vi "Wait on Integer Runtime Test.vi"() -> ()   [LabVIEW 2015, in "Wait on Integer Tests.lvlib"]
uses:
  Wait on Integer Tests.lvlib
  Config/Wait On Integer Config.lvclass
  classes/Step/Execution/StepState.ctl
  classes/Step/Execution/Step Status.ctl
  classes/Step/Execution/Step Flow Control.ctl
  <vilib>/NI/Tag Bus/tag/Data Type.ctl
  <vilib>/NI/Tag Bus Module Framework/channel/channel classification.ctl
  Config/Wait On Integer Config.lvclass/Wait On Integer Config.ctl
  <vilib>/NI/Tag Bus/tag/tag descriptor.lvclass/tag descriptor.ctl
  <vilib>/NI/Tag Bus/table/data polymorphs/write one/write U32.vi
  Config/Write Wait On Integer Event.vi
  Config/Write Target Integer.vi
  Config/Write Timeout.vi
  <vilib>/NI/Tag Bus/tag/read tag name.vi
  <vilib>/NI/Tag Bus/tag/read data type.vi
  <vilib>/NI/Tag Bus/dictionary/locate tag.vi
  classes/Step/Execution/Step.lvclass
  <vilib>/NI/Tag Bus Module Framework/channel/TBM channel.lvclass
  <vilib>/NI/Tag Bus/table/data table.lvlib
  <vilib>/NI/Tag Bus/dictionary/data dictionary.lvclass
  <vilib>/NI/Tag Bus/tag/tag descriptor.lvclass
panel:
  out "error out":errorcluster
  in  "Current Integer":u32
  out "Results":bool[](array[boolean])
  in  "Timeout":i32
  in  "Target Integer":i32
  # "Step State\n\nFlow Control\n\nJump Index\n\nDone"
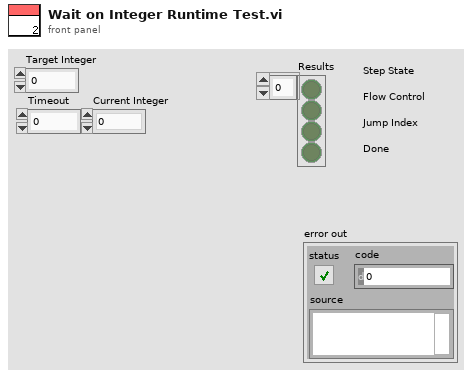
[diagram p1: front panel]
types:
  T1 = typedef "TBM channel.lvclass/channel classification.ctl" = enum16{"input data", "output data", "processing parameter", "processing result"}
  T2 = typedef "tag bus.lvlib/tag descriptor.lvclass/Data Type.ctl" = enum16{"Double", "Single", "I64", "I32", "I16", "I8", "U64", "U32", "U16", "U8", "Boolean", "String", "Array of Double", "Array of Single", "Array of I64", "Array of I32", "Array of I16", "Array of I8", "Array of U64", "Array of U32", "Array of U16", "Array of U8", "Array of Boolean", "Array of String"}
  T3 = typedef "Step.lvclass/Step Status.ctl" = enum16{"Start", "Passed", "Failed", "Error", "Done", "Terminated", "Skipped", "Running"}
  T4 = typedef "Step.lvclass/StepState.ctl" = cluster{"Step State":T3, "Flow Control":T5, "Jump Index":i32, "Done":bool}
  T5 = typedef "Step.lvclass/Step Flow Control.ctl" = enum16{"Next Step", "Jump"}
  T6 = typedef "TBM channel.lvclass/data tables.ctl" = cluster{"input data":T7, "processing parameter":T7, "processing result":T7, "output data":T7}
  T7 = typedef "tag bus.lvlib/dictionary table pair.ctl" = cluster{"data dictionary":refnum<class "data dictionary.lvclass">, "data table":T8}
  T8 = typedef "tag bus.lvlib/data table.lvlib/data table.ctl" = cluster{"Double":dbl[], "Single":sgl[], "I64":i64[], "I32":i32[], "I16":i16[], "I8":i8[], "U64":u64[], "U32":u32[], "U16":u16[], "U8":u8[], "Boolean":bool[], "String":string[], "Array of Double":cluster{"DBL Array":dbl[]}[], "Array of Single":cluster{"SGL Array":sgl[]}[], "Array of I64":cluster{"I64 Array":i64[]}[], "Array of I32":cluster{"I32 Array":i32[]}[], "Array of I16":cluster{"I16 Array":i16[]}[], "Array of I8":cluster{"I8 Array":i8[]}[], "Array of U64":cluster{"U64 Array":u64[]}[], "Array of U32":cluster{"U32 Array":u32[]}[], "Array of U16":cluster{"U16 Array":u16[]}[], "Array of U8":cluster{"U8 Array":u8[]}[], "Array of Boolean":cluster{"Boolean Array":bool[]}[], "Array of String":cluster{"String Array":string[]}[]}
  T9 = cluster{"Step State":bool, "Flow Control":bool, "Jump Index":bool, "Done":bool}
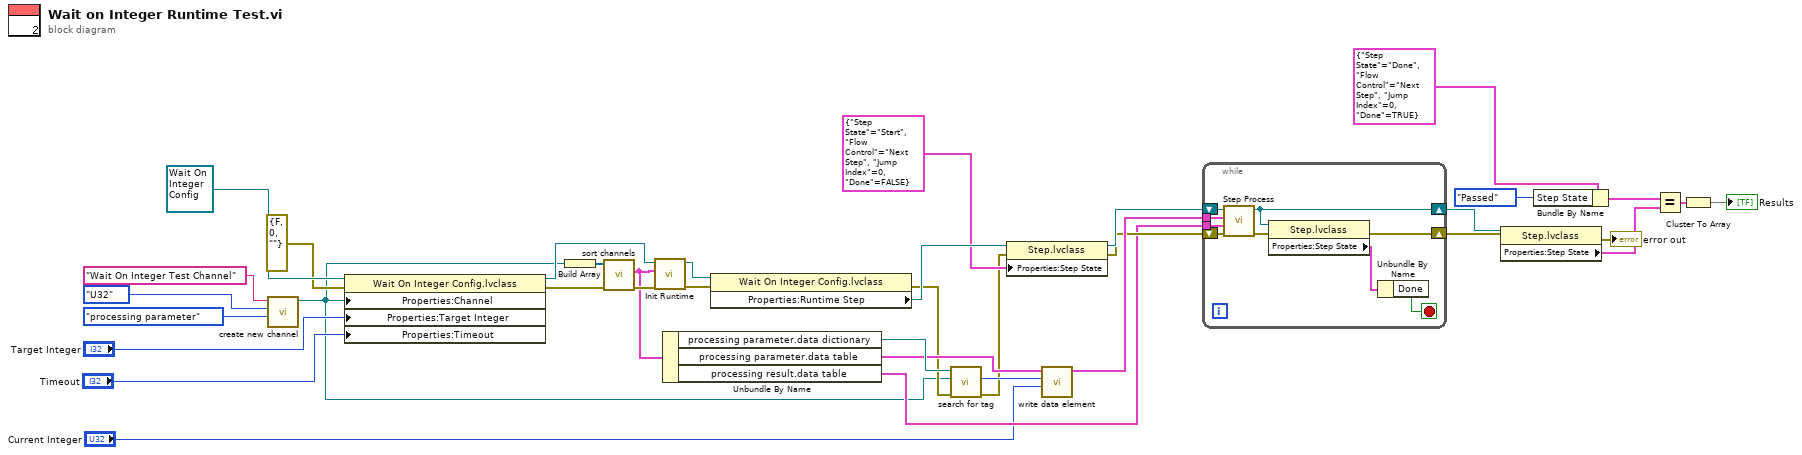
[diagram p0: block diagram]
diagram:
  n1 = call <vilib>:"create new channel.vi"("channel classification"=channel_classification."processing parameter", "data type"=Data_Type."U32", "channel name"="Wait On Integer Test Channel") -> ("channel"=w5:refnum<class "TBM channel.lvclass">)  [unwired: 8 in]
  n2 = property class="Wait On Integer Config.lvclass"(reference=refnum<class "Wait On Integer Config.lvclass"> refnum ("Wait On Integer Step Config.lvclass"), error in=errorcluster {"status"=FALSE, "code"=0, "source"=""} ("error in (no error)"), "Properties:Channel"=w5, "Properties:Target Integer"="Target Integer", "Properties:Timeout"="Timeout") -> (reference out=w31:refnum<class "Wait On Integer Config.lvclass">, error out=w32:errorcluster)
  n3 = Build Array(w5) -> (w33:refnum<class "TBM channel.lvclass">[])
  n4 = call <vilib>:"sort channels.vi"("error in"=w32, "channels in"=w33) -> ("error out"=w30:errorcluster, "data allocations"=w2:T6)  [unwired: 7 in, 1 out]
  n5 = call-dynamic "Init Runtime.vi"("error in (no error)"=w30, "data allocations"=w2, "Wait On Integer Step Config in"=w31) -> ("error out"=w28:errorcluster, "Wait On Integer Step Config out"=w29:refnum<class "Wait On Integer Config.lvclass">)  [unwired: 6 in, 1 out]
  n6 = Unbundle By Name(w2) -> ("processing parameter.data dictionary"=w26:refnum<class "data dictionary.lvclass">, "processing parameter.data table"=w23:T8, "processing result.data table"=w16:T8)
  n7 = property class="Wait On Integer Config.lvclass"(reference=w29, error in=w28) -> (error out=w18:errorcluster, "Properties:Runtime Step"=w25:refnum<class "Step.lvclass">)  [unwired: 1 out]
  n8 = call <vilib>:"search for tag.vi"("error in"=w18, "system tag"=w5, "data dictionary in"=w26) -> ("error out"=w6:errorcluster, "index"=w22:i32)  [unwired: 6 in, 1 out]
  n9 = property class="Step.lvclass"(reference=w25, error in=w6, "Properties:Step State"=T4 {"Step State"=enum."Start", "Flow Control"=enum."Next Step", "Jump Index"=0, "Done"=FALSE} ("Step State")) -> (reference out=w21:refnum<class "Step.lvclass">, error out=w17:errorcluster)
  n10 = call-poly <vilib>:"write data element.vi"("value"="Current Integer", "index"=w22, "data table in"=w23) -> ("data table out"=w20:T8)  [unwired: 8 in]
  n11 = while {
    tunnel: w20 -> [w44]
    tunnel: w16 -> [w42]
    shift-right: [w41] -> w19
    shift-left: w21 -> [w45]
    shift-right: [w39] -> w15
    shift-left: w17 -> [w43]
    stop <- w37 stop-if-true
    n12 = call-dynamic "Step Process.vi"("error in (no error)"=w43, "result allocation"=w42, "parameters"=w44, "Step in"=w45) -> ("error out"=w40:errorcluster, "Step out"=w41:refnum<class "Step.lvclass">)  [unwired: 4 in, 2 out]
    n13 = property class="Step.lvclass"(reference=w41, error in=w40) -> (error out=w39:errorcluster, "Properties:Step State"=w38:T4)  [unwired: 1 out]
    n14 = Unbundle By Name(w38) -> ("Done"=w37:bool)
  }
  n15 = property class="Step.lvclass"(reference=w19, error in=w15) -> (error out=→"error out":errorcluster, "Properties:Step State"=w10:T4)  [unwired: 1 out]
  n16 = Bundle By Name(cluster=T4 {"Step State"=enum."Done", "Flow Control"=enum."Next Step", "Jump Index"=0, "Done"=TRUE} ("Step State"), "Step State"=Step_Status."Passed") -> (w11:T4)
  n17 = Equal?(x=w11, y=w10) -> (x = y?=w9:T9)
  n18 = Cluster To Array(cluster=w9) -> (array=→"Results":bool[])
